vi "R1SBRControl_Status.vi"(7 "LabVIEW Web Service Request":refnum<class "Web Request.lvclass">) -> (0 "error out":errorcluster, 3 "SBRData":T1)   [LabVIEW 2016]
uses:
  Controls/R7SBR_SetParams.ctl
  R1Controls/R7SBR_Status.ctl
  <vilib>/wsapi/Web Request.lvclass
panel:
  # "Use the Web Service Request input terminal to call the VIs on the Web Services palette. Do not remove it from the connector pane unless you don't need access to the palette."
  # "Each additional control wired to the connector pane will be available as an input in the URL. To include an indicator in terminal-mode output (the default setting), it must also be wired to the connector pane."
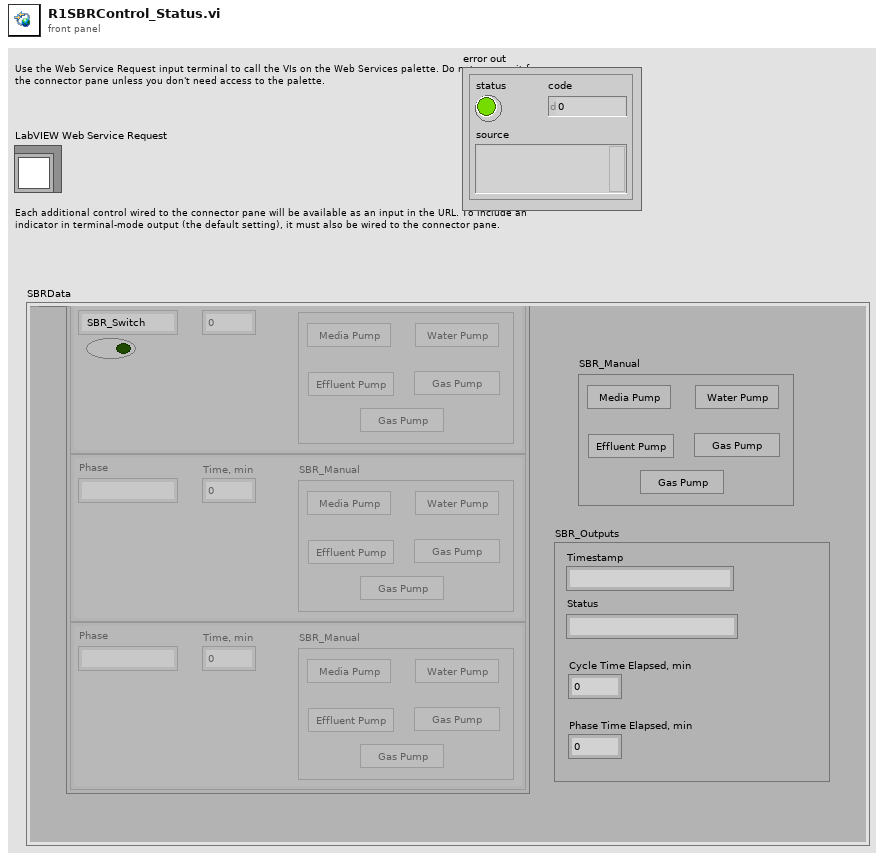
[diagram p1: front panel]
types:
  T1 = typedef "R7SBR_Status.ctl" = cluster{"SBR_Switch":bool, "SBR_SetParams":T2, "SBR_Manual":cluster{"Media Pump":bool, "Water Pump":bool, "Effluent Pump":bool, "Release Valve":bool, "Gas Pump":bool}, "SBR_Outputs":cluster{"Cycle Time Elapsed, min":dbl, "Phase Time Elapsed, min":dbl, "Timestamp":string, "Status":string}}
  T2 = typedef "R7SBR_SetParams.ctl" = cluster{"Phase":string, "Time, min":dbl, "SBR_Manual":cluster{"Media Pump":bool, "Water Pump":bool, "Effluent Pump":bool, "Release Valve":bool, "Gas Pump":bool}}[]
  T3 = cluster{"Media Pump":bool, "Water Pump":bool, "Effluent Pump":bool, "Release Valve":bool, "Gas Pump":bool}
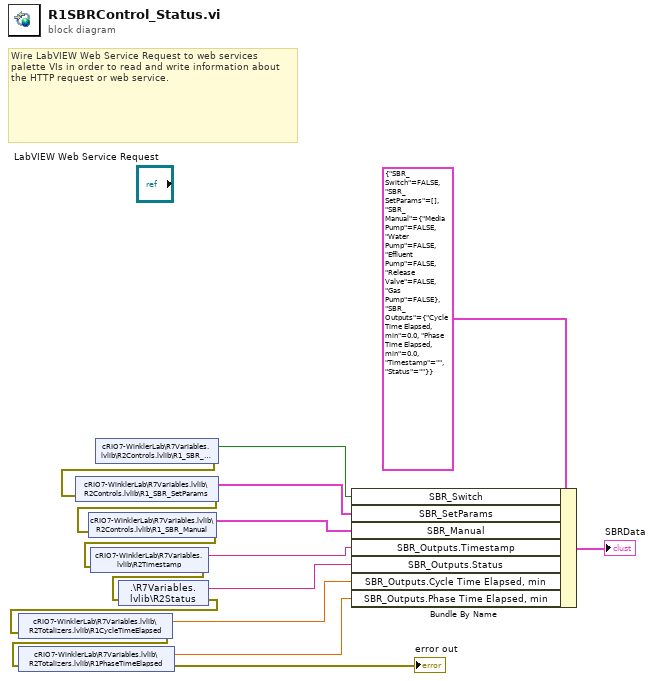
[diagram p0: block diagram]
diagram:
  # "Wire LabVIEW Web Service Request to web services palette VIs in order to read and write information about the HTTP request or web service."
  n1 = shared-variable "cRIO7-WinklerLab\\R7Variables.lvlib\\R2Controls.lvlib\\R1_SBR_Switch"() -> (w15:bool, error out=w11:errorcluster)  [unwired: 1 in]
  n2 = shared-variable "cRIO7-WinklerLab\\R7Variables.lvlib\\R2Controls.lvlib\\R1_SBR_SetParams"(error in=w11) -> (w16:T2, error out=w4:errorcluster)
  n3 = shared-variable "cRIO7-WinklerLab\\R7Variables.lvlib\\R2Controls.lvlib\\R1_SBR_Manual"(error in=w4) -> (w2:T3, error out=w3:errorcluster)
  n4 = shared-variable "cRIO7-WinklerLab\\R7Variables.lvlib\\R2Timestamp"(error in=w3) -> (w8:string, error out=w6:errorcluster)
  n5 = shared-variable ".\\R7Variables.lvlib\\R2Status"(error in=w6) -> (w7:string, error out=w10:errorcluster)
  n6 = shared-variable "cRIO7-WinklerLab\\R7Variables.lvlib\\R2Totalizers.lvlib\\R1CycleTimeElapsed"(error in=w10) -> (w14:dbl, error out=w5:errorcluster)
  n7 = shared-variable "cRIO7-WinklerLab\\R7Variables.lvlib\\R2Totalizers.lvlib\\R1PhaseTimeElapsed"(error in=w5) -> (w13:dbl, error out=→"error out":errorcluster)
  n8 = Bundle By Name(cluster=T1 {"SBR_Switch"=FALSE, "SBR_SetParams"=[], "SBR_Manual"={"Media Pump"=FALSE, "Water Pump"=FALSE, "Effluent Pump"=FALSE, "Release Valve"=FALSE, "Gas Pump"=FALSE}, "SBR_Outputs"={"Cycle Time Elapsed, min"=0.0, "Phase Time Elapsed, min"=0.0, "Timestamp"="", "Status"=""}} ("SBRData"), "SBR_Switch"=w15, "SBR_SetParams"=w16, "SBR_Manual"=w2, "SBR_Outputs.Timestamp"=w8, "SBR_Outputs.Status"=w7, "SBR_Outputs.Cycle Time Elapsed, min"=w14, "SBR_Outputs.Phase Time Elapsed, min"=w13) -> (→"SBRData":T1)
